vi "Configure CAN STP.vi"(6 "Log Data?":bool=TRUE, 8 "error in":errorcluster, 9 "Socket No":u16=1, 10 "STP Data in":T3={"ECU CAN Port"="CAN1", "CMD"=130, "CAN Write Data"=[], "Response Decoder"=enum."String", "String"={"Start Index"=0, "Length"=-1}, "Number"={"MSB Index"=0, "LSB Index"=1}, "Boolean"={"Index"=0, "Bool"={"7"=FALSE, "6"=FALSE, "5"=FALSE, "4"=FALSE, "3"=FALSE, "2"=FALSE, "1"=FALSE, "0"=FALSE, "7 Enabled"=FALSE, "6 Enabled"=FALSE, "5 Enabled"=FALSE, "4 Enabled"=FALSE, "3 Enabled"=FALSE, "2 Enabled"=FALSE, "1 Enabled"=FALSE, "0 Enabled"=FALSE}}} {"CMD" items=["TSW_VERSION(130)"=130, "WAIT_EVENT(132)"=132, "SEQUENCER(133)"=133, "TSW_RESET(150)"=150, "CONFIG_ECU(151)"=151, "TEST_CORE (152)"=152, "TEST_WATCHDOG (153)"=153, "TEST_MONITORING (154)"=154, "READ_MEMORY (162)"=162, "WRITE_ERASE_MEMORY (164)"=164, "COMM_EXTERNAL (190)"=190, "COMM_INTERNAL (195)"=195, "GET_ANALOG_INPUT (210)"=210, "GET_DIGITAL_INPUT (211)"=211, "GET_FREQUENCY_INPUT (212)"=212, "TEST_INPUT_STRUCTURE (214)"=214, "GENERATE_OUTPUT_SIGNAL (220)"=220, "GENERATE_SYNCHRONIZED_OUTPUT_SIGNALS (221)"=221, "eDCU_Specific (250)"=250]; "CAN Write Data" format="%.0x"}) -> (0 "error out":errorcluster, 1 "STP Error":T1, 2 "STP Data Out":T2, 3 "Report Text":string)   [LabVIEW 2023]
uses:
  HardwareAbstractionLayer_LVOOP/CAN/CAN Application Protocols/STP Protocol_class/STP Protocol.lvclass
  HardwareAbstractionLayer_LVOOP/CAN/CAN Application Protocols/STP Protocol_class/Ctrls/STP CMD.ctl
  HardwareAbstractionLayer_LVOOP/CAN/CAN Application Protocols/STP Protocol_class/Ctrls/STP Input Data.ctl
  <vilib>/xnet/xnet.llb/XNET Control Scope.ctl
  HardwareAbstractionLayer_LVOOP/CAN/CAN Lib/CAN_class/Ctrls/CAN Init Ctrl.ctl
  HardwareAbstractionLayer_LVOOP/CAN/CAN Lib/CAN_class/CAN.lvclass
  HardwareAbstractionLayer_LVOOP/Database/Database.lvclass
  Teststand Steptypes/CAN/STP/Steptypes/Control/STP Out Data.ctl
  Teststand Steptypes/LTT_TeststandSteptypes.lvlib
  Teststand Steptypes/CAN/STP/Steptypes/Control/STP Data.ctl
  HardwareAbstractionLayer_LVOOP/CAN/CAN Application Protocols/STP Protocol_class/Ctrls/STP Error Cluster.ctl
panel:
  # "Help : the index will choose the one element in an array and compare its true or false"
  # "Bit"
  # "Value"
  # "Enabled"
  # "Help : if the LSB index is -1 then it will take only MSB value"
  # "Help : if length -1 then it will take the entire array"
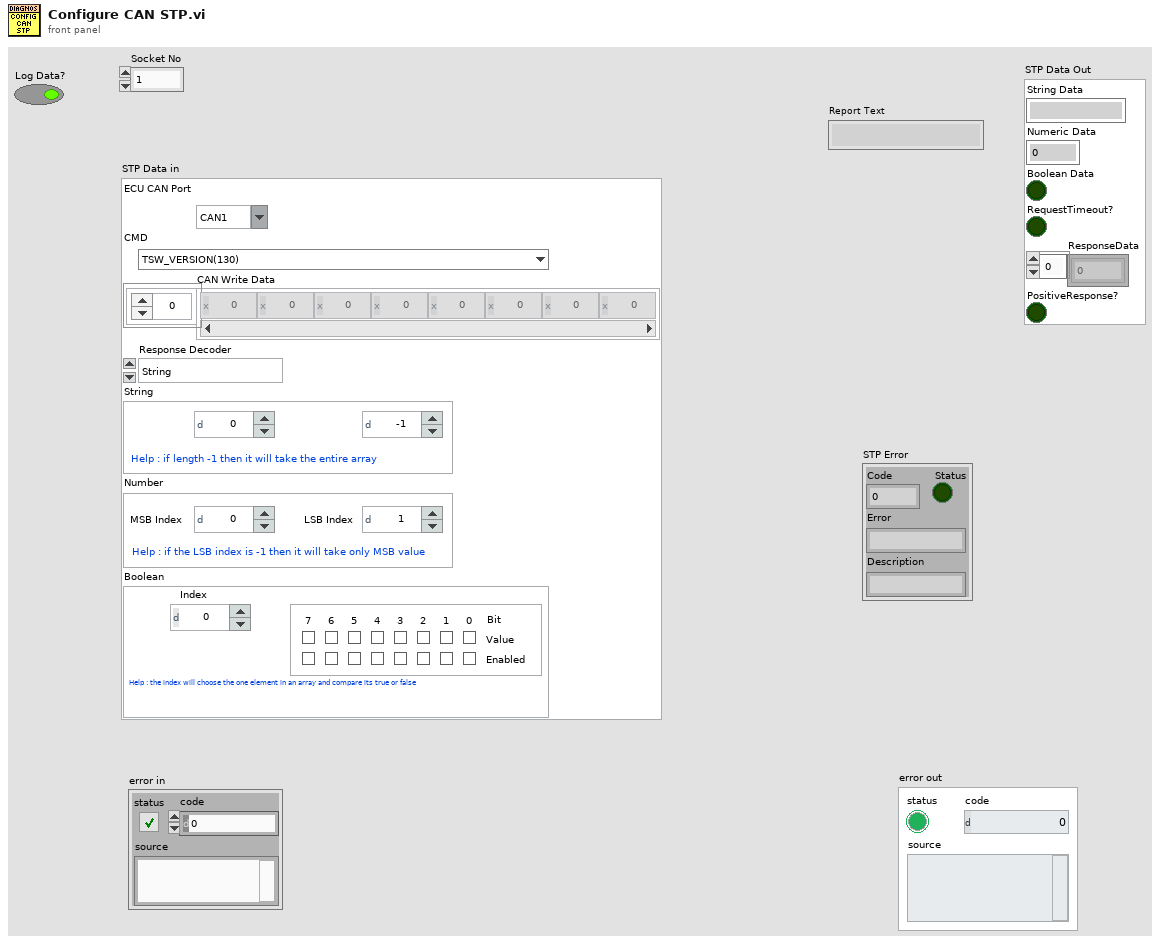
[diagram p1: front panel]
types:
  T1 = typedef "HardwareAbstractionLayer_LVOOP.lvlib/CAN Application Protocols Lib.lvlib/STP Protocol.lvclass/STP Error Cluster.ctl" = cluster{"Status":bool, "Code":u8, "Error":string, "Description":string}
  T2 = typedef "LTT_TeststandSteptypes.lvlib/STP Out Data.ctl" = cluster{"String Data":string, "Numeric Data":dbl, "Boolean Data":bool, "RequestTimeout?":bool, "ResponseData":u8[], "PositiveResponse?":bool}
  T3 = typedef "LTT_TeststandSteptypes.lvlib/STP Data.ctl" = cluster{"ECU CAN Port":string, "CMD":T4, "CAN Write Data":u8[], "Response Decoder":enum16{"String", "Number", "Boolean"}, "String":cluster{"Start Index":i32, "Length":i32}, "Number":cluster{"MSB Index":i32, "LSB Index":i32}, "Boolean":cluster{"Index":i32, "Bool":cluster{"7":bool, "6":bool, "5":bool, "4":bool, "3":bool, "2":bool, "1":bool, "0":bool, "7 Enabled":bool, "6 Enabled":bool, "5 Enabled":bool, "4 Enabled":bool, "3 Enabled":bool, "2 Enabled":bool, "1 Enabled":bool, "0 Enabled":bool}}}
  T4 = typedef "HardwareAbstractionLayer_LVOOP.lvlib/CAN Application Protocols Lib.lvlib/STP Protocol.lvclass/STP CMD.ctl" = u8
  T5 = typedef "HardwareAbstractionLayer_LVOOP.lvlib/CAN HAL Lib.lvlib/CAN.lvclass/CAN Init Ctrl.ctl" = cluster{"XNET Interface":refnum<k21>, "Baud Rate":u64, "CAN:Termination":u32, "Echo Transmit?":bool, "scope (normal)":T6}
  T6 = typedef "XNET Control Scope.ctl" = u32
  T7 = typedef "HardwareAbstractionLayer_LVOOP.lvlib/CAN Application Protocols Lib.lvlib/STP Protocol.lvclass/STP Input Data.ctl" = cluster{"TxID":u32, "RxID":u32, "CMD":T4, "RQ Data":u8[], "+veResponseCode":u8, "ResponseTimeout (S)":dbl}
  T8 = typedef "HardwareAbstractionLayer_LVOOP.lvlib/CAN Application Protocols Lib.lvlib/STP Protocol.lvclass/STP Output Data.ctl" = cluster{"ResponseData":u8[], "ResponseData(ASCII)":string, "PositiveResponse?":bool, "STP Error":T1}
  T9 = cluster{"7":bool, "6":bool, "5":bool, "4":bool, "3":bool, "2":bool, "1":bool, "0":bool, "7 Enabled":bool, "6 Enabled":bool, "5 Enabled":bool, "4 Enabled":bool, "3 Enabled":bool, "2 Enabled":bool, "1 Enabled":bool, "0 Enabled":bool}
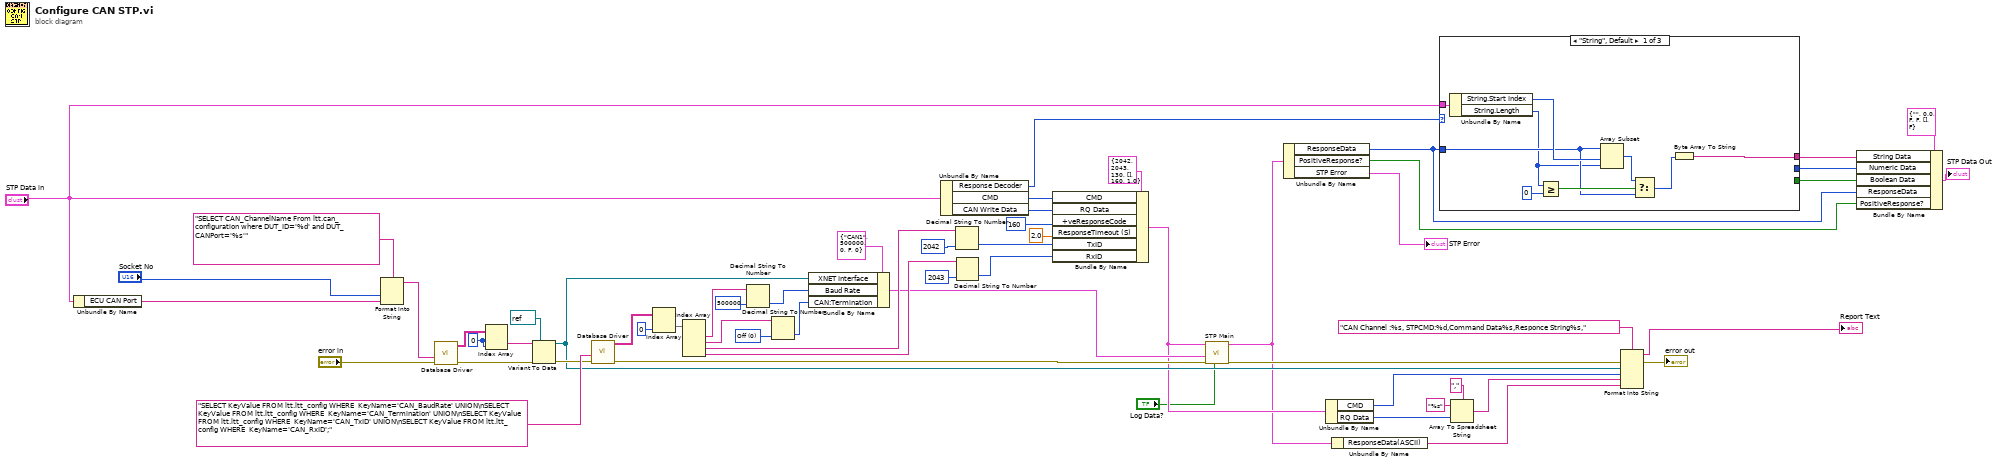
[diagram p0: block diagram]
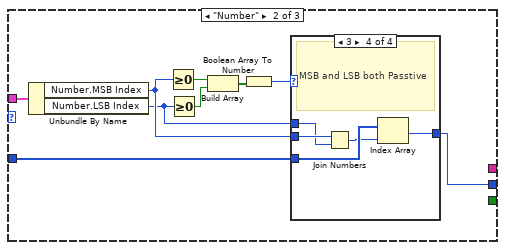
[diagram p2: hidden frame]
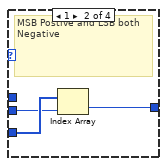
[diagram p4: hidden frame]
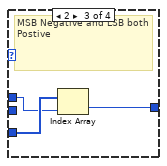
[diagram p5: hidden frame]
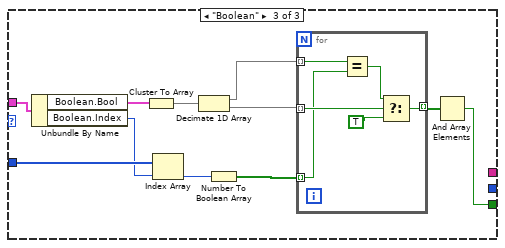
[diagram p6: hidden frame]
diagram:
  w35 = u32 0 items=["Off", "On"] ("CAN:Termination")
  w48 = 0 ("index (row)")
  n1 = Unbundle By Name("STP Data in") -> ("ECU CAN Port"=w50:string)
  n2 = Format Into String(format string="SELECT CAN_ChannelName From ltt.can_configuration where DUT_ID='%d' and DUT_CANPort='%s'" ("SQL query"), "Socket No", w50) -> (resulting string=w52:string)  [unwired: 2 in, 1 out]
  n3 = call "Database Driver.vi"("error in"="error in", "SQL query"=w52) -> ("error out"=w45:errorcluster, "data"=w49:string[][])  [unwired: 6 in, 2 out]
  n4 = Index Array(array=w49, index (row)=w48, index (col)=w48) -> (element=w46:string)
  n5 = Variant To Data(error in=w45, type=refnum<k21> refnum ("XNET Interface"), Variant=w46) -> (data=w15:refnum<k21>, error out=w43:errorcluster)
  n6 = call "Database Driver.vi"("error in"=w43, "SQL query"="SELECT KeyValue FROM ltt.ltt_config WHERE  KeyName='CAN_BaudRate' UNION\nSELECT KeyValue FROM ltt.ltt_config WHERE  KeyName='CAN_Termination' UNION\nSELECT KeyValue FROM ltt.ltt_config WHERE  KeyName='CAN_TxID' UNION\nSELECT KeyValue FROM ltt.ltt_config WHERE  KeyName='CAN_RxID';") -> ("error out"=w26:errorcluster, "data"=w42:string[][])  [unwired: 6 in, 2 out]
  n7 = Index Array(array=w42, index (col)=0 ("disabled index (col)")) -> (element=w40:string[])  [unwired: 1 in]
  n8 = Index Array(array=w40) -> (element #1=w39:string, element #2=w36:string, element #3=w33:string, element #4=w32:string)  [unwired: 4 in]
  n9 = Decimal String To Number(string=w39, default (0L)=u64 500000 ("Baud Rate")) -> (number=w37:u64)  [unwired: 1 in, 1 out]
  n10 = Decimal String To Number(string=w36, default (0L)=w35) -> (number=w34:u32)  [unwired: 1 in, 1 out]
  n11 = Bundle By Name(cluster=T5 {"XNET Interface"="CAN1", "Baud Rate"=500000, "CAN:Termination"=0, "Echo Transmit?"=FALSE, "scope (normal)"=0} ("CAN Init Data"), "XNET Interface"=w15, "Baud Rate"=w37, "CAN:Termination"=w34) -> (w27:T5)
  n12 = Unbundle By Name("STP Data in") -> ("Response Decoder"=w12:enum16{"String", "Number", "Boolean"}, "CMD"=w58:T4, "CAN Write Data"=w57:u8[])
  n13 = Decimal String To Number(string=w33, default (0L)=u32 2042 ("TxID")) -> (number=w31:u32)  [unwired: 1 in, 1 out]
  n14 = Decimal String To Number(string=w32, default (0L)=u32 2043 ("TxID")) -> (number=w28:u32)  [unwired: 1 in, 1 out]
  n15 = Bundle By Name(cluster=T7 {"TxID"=2042, "RxID"=2043, "CMD"=130, "RQ Data"=[], "+veResponseCode"=160, "ResponseTimeout (S)"=1.0} ("STP Input Data"), "CMD"=w58, "RQ Data"=w57, "+veResponseCode"=u8 160, "ResponseTimeout (S)"=2.0, "TxID"=w31, "RxID"=w28) -> (w11:T7)
  n16 = call "STP Main.vi"("Log Data?"="Log Data?", "error in (no error)"=w26, "CAN Init Data"=w27, "STP Input Data"=w11) -> ("error out"=w14:errorcluster, "STP Output Data"=w4:T8)  [unwired: 5 in, 1 out]
  n17 = Unbundle By Name(w4) -> ("ResponseData"=w20:u8[], "PositiveResponse?"=w18:bool, "STP Error"=→"STP Error":T1)
  n18 = Unbundle By Name(w11) -> ("CMD"=w10:T4, "RQ Data"=w9:u8[])
  n19 = Unbundle By Name(w4) -> ("ResponseData(ASCII)"=w3:string)
  n20 = case shown="\"String\", Default" w12 {
    tunnel: w20 -> [w61 w72 w96]
    tunnel: "STP Data in" -> [w68 w77 w99]
    tunnel: [w66 _ _] -> w23
    tunnel: [_ w69 _] -> w22
    tunnel: [_ _ w89] -> w21
    frame "String", Default {
      n21 = Unbundle By Name(w68) -> ("String.Start Index"=w67:i32, "String.Length"=w60:i32)
      n22 = Greater Or Equal?(x=w60, y=0) -> (x >= y?=w65:bool)
      n23 = Array Subset(array=w61, index=w67, length=w60) -> (w63:u8[])
      n24 = Select(t=w63, s=w65, f=w61) -> (s? t:f=w62:u8[])
      n25 = Byte Array To String(unsigned byte array=w62) -> (string=w66:string)
    }
    frame "Number" {
      n26 = Unbundle By Name(w77) -> ("Number.MSB Index"=w71:i32, "Number.LSB Index"=w70:i32)
      n27 = Greater Or Equal To 0?(x=w71) -> (x >= 0?=w76:bool)
      n28 = Greater Or Equal To 0?(x=w70) -> (x >= 0?=w75:bool)
      n29 = Build Array(w76, w75) -> (w74:bool[])
      n30 = Boolean Array To Number(Boolean array=w74) -> (number=w73:u32)
      n31 = case shown="3" w73 {
        tunnel: w72 -> [_ w80 w83 w88]
        tunnel: w71 -> [_ w79 _ w86]
        tunnel: w70 -> [_ _ w81 w85]
        tunnel: [_ w78 w82 w87] -> w69
        frame 0, Default {
          # "MSB and LSB both Negative"
        }
        frame 1 {
          # "MSB Postive and LSB both Negative"
          n32 = Index Array(array=w80, index=w79) -> (element=w78:u8)
        }
        frame 2 {
          # "MSB Negative and LSB both Postive"
          n33 = Index Array(array=w83, index=w81) -> (element=w82:u8)
        }
        frame 3 {
          # "MSB and LSB both Passtive"
          n34 = Join Numbers(hi=w86, lo=w85) -> ((hi.lo)=w84:u64)
          n35 = Index Array(array=w88, index=w84) -> (element=w87:u8)
        }
      }
    }
    frame "Boolean" {
      n36 = Unbundle By Name(w99) -> ("Boolean.Bool"=w98:T9, "Boolean.Index"=w95:i32)
      n37 = Cluster To Array(cluster=w98) -> (array=w97:bool[])
      n38 = Index Array(array=w96, index=w95) -> (element=w94:u8)
      n39 = Decimate 1D Array(w97) -> (w92:bool[], w91:bool[])
      n40 = Number To Boolean Array(number=w94) -> (Boolean array=w93:bool[])
      n41 = for {
        tunnel: w93 -> [w103] mode=indexing
        tunnel: w92 -> [w104] mode=indexing
        tunnel: w91 -> [w105] mode=indexing
        tunnel: [w100] -> w90 mode=indexing
        n42 = Equal?(x=w104, y=w103) -> (x = y?=w102:bool)
        n43 = Select(t=w102, s=w105, f=TRUE) -> (s? t:f=w100:bool)
      }
      n44 = And Array Elements(Boolean array=w90) -> (logical AND=w89:bool)
    }
  }
  n45 = Array To Spreadsheet String(delimiter (Tab)=",", array=w9, 3:"%s" ("format string")) -> (spreadsheet string=w7:string)
  n46 = Format Into String(format string="CAN Channel :%s, STPCMD:%d,Command Data%s,Responce String%s,", error in=w14, w15, w10, w7, w3) -> (resulting string=→"Report Text":string, error out=→"error out":errorcluster)  [unwired: 1 in]
  n47 = Bundle By Name(cluster=T2 {"String Data"="", "Numeric Data"=0.0, "Boolean Data"=FALSE, "RequestTimeout?"=FALSE, "ResponseData"=[], "PositiveResponse?"=FALSE} ("STP Data Out"), "String Data"=w23, "Numeric Data"=w22, "Boolean Data"=w21, "ResponseData"=w20, "PositiveResponse?"=w18) -> (→"STP Data Out":T2)
